vi "Gen Status Display.vi"(8 "Error In":errorcluster, 11 "MSI Data":T1 {"Converter Faults 2" format="%016b"; "Converter Alarms 2" format="%016b"; "Converter Faults 1" format="%016b"; "Converter Alarms 1" format="%016b"; "Solar Faults" format="%016b"; "ES Rack 10 Alarms" format="%016b"; "ES Rack 9 Alarms" format="%016b"; "ES Rack 8 Alarms" format="%016b"; "ES Rack 7 Alarms" format="%016b"; "ES Rack 6 Alarms" format="%016b"; "ES Rack 5 Alarms" format="%016b"; "ES Rack 4 Alarms" format="%016b"; "ES Rack 3 Alarms" format="%016b"; "ES Rack 2 Alarms" format="%016b"; "ES Rack 1 Alarms" format="%016b"; "ES System Alarms" format="%016b"; "System Faults" format="%016b"; "ES Rack 10 Faults" format="%016b"; "Es Rack 9 Faults" format="%016b"; "ES Rack 8 Faults" format="%016b"; "ES Rack 7 Faults" format="%016b"; "ES Rack 6 Faults" format="%016b"; "ES Rack 5 Faults" format="%016b"; "ES Rack 4 Faults" format="%016b"; "ES Rack 3 Faults" format="%016b"; "ES Rack 2 Faults" format="%016b"; "ES Rack 1 Faults" format="%016b"; "ES System Faults" format="%016b"; "System Status" format="%016b"; "Controller Faults" format="%016b"}) -> (0 "Error Out":errorcluster, 3 "Gen Status Data":bool[](array[boolean]))   [LabVIEW 2014]
uses:
  Controls/Modbus Status Interface Data MOD2.ctl
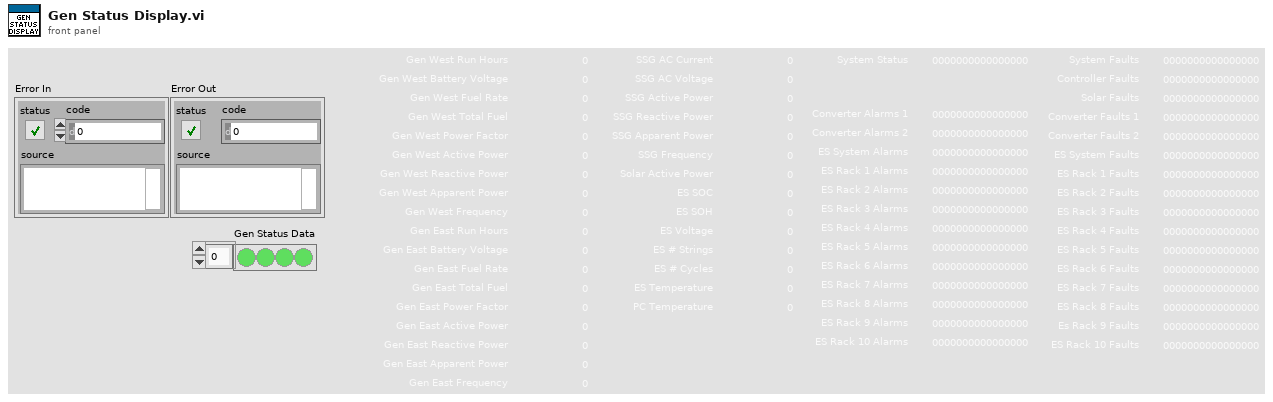
[diagram p1: front panel]
types:
  T1 = typedef "Modbus Status Interface Data MOD2.ctl" = cluster{"SSG AC Current":i16, "SSG AC Voltage":i16, "SSG Active Power":i16, "SSG Reactive Power":i16, "SSG Apparent Power":i16, "SSG Frequency":i16, "ES SOC":i16, "ES SOH":i16, "ES Voltage":i16, "ES # Strings":i16, "ES # Cycles":i16, "ES Temperature":i16, "PC Temperature":i16, "Solar Active Power":i16, "Gen West Run Hours":i16, "Gen West Battery Voltage":i16, "Gen West Fuel Rate":i16, "Gen West Total Fuel":i16, "Gen West Power Factor":i16, "Gen West Active Power":i16, "Gen West Reactive Power":i16, "Gen West Apparent Power":i16, "Gen West Frequency":i16, "Gen East Run Hours":i16, "Gen East Battery Voltage":i16, "Gen East Fuel Rate":i16, "Gen East Total Fuel":i16, "Gen East Power Factor":i16, "Gen East Active Power":i16, "Gen East Reactive Power":i16, "Gen East Apparent Power":i16, "Gen East Frequency":i16, "Converter Version":i16, "Controller Version":i16, "System Status":i16, "System Faults":i16, "Controller Faults":i16, "ES System Faults":i16, "ES System Alarms":i16, "Converter Faults 1":i16, "Converter Faults 2":i16, "Converter Alarms 1":i16, "Converter Alarms 2":i16, "Solar Faults":i16, "ES Rack 1 Faults":i16, "ES Rack 2 Faults":i16, "ES Rack 3 Faults":i16, "ES Rack 4 Faults":i16, "ES Rack 5 Faults":i16, "ES Rack 6 Faults":i16, "ES Rack 7 Faults":i16, "ES Rack 8 Faults":i16, "Es Rack 9 Faults":i16, "ES Rack 10 Faults":i16, "ES Rack 1 Alarms":i16, "ES Rack 2 Alarms":i16, "ES Rack 3 Alarms":i16, "ES Rack 4 Alarms":i16, "ES Rack 5 Alarms":i16, "ES Rack 6 Alarms":i16, "ES Rack 7 Alarms":i16, "ES Rack 8 Alarms":i16, "ES Rack 9 Alarms":i16, "ES Rack 10 Alarms":i16}
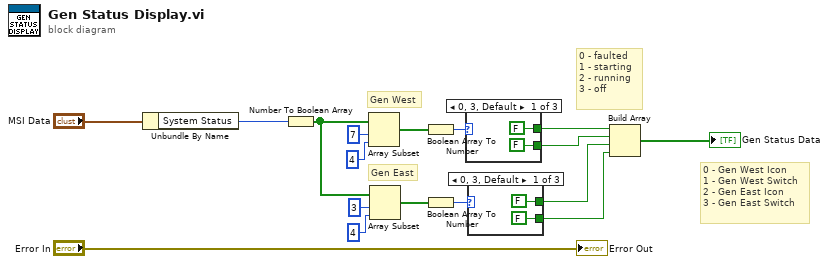
[diagram p0: block diagram]
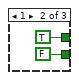
[diagram p2: hidden frame]
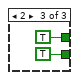
[diagram p3: hidden frame]
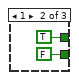
[diagram p4: hidden frame]
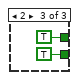
[diagram p5: hidden frame]
diagram:
  # "Gen East"
  # "Gen West"
  # "0 - Gen West Icon\n1 - Gen West Switch\n2 - Gen East Icon\n3 - Gen East Switch"
  # "0 - faulted\n1 - starting\n2 - running \n3 - off"
  n1 = Unbundle By Name("MSI Data") -> ("System Status"=w3:i16)
  n2 = Number To Boolean Array(number=w3) -> (Boolean array=w5:bool[])
  n3 = Array Subset(array=w5, index=7, length=4) -> (w8:bool[])
  n4 = Array Subset(array=w5, index=3, length=4) -> (w4:bool[])
  n5 = Boolean Array To Number(Boolean array=w8) -> (number=w2:u8)
  n6 = Boolean Array To Number(Boolean array=w4) -> (number=w1:u8)
  n7 = case shown="0, 3, Default" w2 {
    tunnel: [FALSE TRUE TRUE] -> w15
    tunnel: [FALSE FALSE TRUE] -> w14
    frame 0, 3, Default {
    }
    frame 1 {
    }
    frame 2 {
    }
  }
  n8 = case shown="0, 3, Default" w1 {
    tunnel: [FALSE TRUE TRUE] -> w13
    tunnel: [FALSE FALSE TRUE] -> w12
    frame 0, 3, Default {
    }
    frame 1 {
    }
    frame 2 {
    }
  }
  n9 = Build Array(w15, w14, w13, w12) -> (→"Gen Status Data":bool[])
  "Error Out" <- "Error In"
